vi "test_DELETE.vi"(11 "NXT":T1={"Hardware"="NXT", "Flattened String"=""}) -> (0 "right(T)/left(F)":bool)   [LabVIEW 2012]
uses:
  <vilib>/NXT/Subs/LVHSConnector.ctl
  <vilib>/NXT/Subs/MotorOutput.ctl
  <vilib>/NXT/Block Support/NXT_InputPort.ctl
  <vilib>/NXT/Dual Mode Library/Motors/MotorOn.vi
  <vilib>/NXT/Dual Mode Library/Motors/MotorReverse.vi
  <vilib>/NXT/Dual Mode Library/Motors/MotorBrake.vi
  <vilib>/NXT/Dual Mode Library/Display/clearDisplay.vi
  <vilib>/NXT/Dual Mode Library/Waits/Wait_Num(msec).vi
  <vilib>/NXT/Dual Mode Library/Sound/Tone.vi
  <vilib>/NXT/Dual Mode Library/Display/drawLine.vi
  <vilib>/NXT/Dual Mode Library/prims/addArrayElements_int.vi
  <vilib>/NXT/Dual Mode Library/prims/rotateArray/rotateArray_int.vi
  <vilib>/NXT/Dual Mode Library/Waits/Wait_Num.vi
  <vilib>/NXT/Dual Mode Library/Display/drawText.vi
  <vilib>/NXT/Dual Mode Library/Display/drawNumber.vi
panel:
  in  "degrees to  rotate":dbl
  out "Array 2":i32[](array[numeric])
types:
  T1 = typedef "LVHSConnector.ctl" = cluster{"Hardware":string, "Flattened String":string}
  T2 = typedef "MotorOutput.ctl" = u8
  T3 = typedef "NXT_InputPort.ctl" = u8
  T4 = cluster{"x-y*floor(x/y)":i32, "Start X":i16, "x-y*floor(x/y)":i32, i16}
  T5 = cluster{"x":i32, "Start X":i16, "x":i32, "Start X":i16}
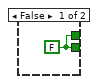
[diagram p2: hidden frame]
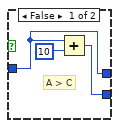
[diagram p3: hidden frame]
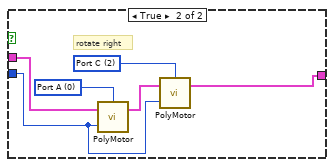
[diagram p5: hidden frame]
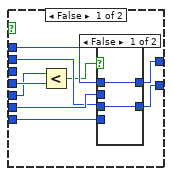
[diagram p16: hidden frame]
diagram:
  w6 = 0
  w9 = T2 5 items=["Port A"=0, "Port B"=1, "Port C"=2, "Ports A & B"=4, "Ports A & C"=5, "Ports B & C"=6, "All Ports"=3] ("Output Port (All Ports)")
  w7 = T2 5 items=["Port A"=0, "Port B"=1, "Port C"=2, "Ports A & B"=4, "Ports A & C"=5, "Ports B & C"=6, "All Ports"=3] ("Output Port (All Ports)")
  w16 = T2 5 items=["Port A"=0, "Port B"=1, "Port C"=2, "Ports A & B"=4, "Ports A & C"=5, "Ports B & C"=6, "All Ports"=3] ("Port (All Ports)")
  w3 = i16 100 ("y")
  (unwired) 2.09 ("Max Value")
  w21 = T2 5 items=["Port A"=0, "Port B"=1, "Port C"=2, "Ports A & B"=4, "Ports A & C"=5, "Ports B & C"=6, "All Ports"=3] ("Port (All Ports)")
  w25 = T2 5 items=["Port A"=0, "Port B"=1, "Port C"=2, "Ports A & B"=4, "Ports A & C"=5, "Ports B & C"=6, "All Ports"=3] ("Port (All Ports)")
  w32 = T2 5 items=["Port A"=0, "Port B"=1, "Port C"=2, "Ports A & B"=4, "Ports A & C"=5, "Ports B & C"=6, "All Ports"=3] ("Port (All Ports)")
  w38 = T2 5 items=["Port A"=0, "Port B"=1, "Port C"=2, "Ports A & B"=4, "Ports A & C"=5, "Ports B & C"=6, "All Ports"=3] ("Port (All Ports)")
  w42 = T2 2 items=["Port A"=0, "Port B"=1, "Port C"=2, "Ports A & B"=4, "Ports A & C"=5, "Ports B & C"=6, "as"=3] ("Output Port (All Ports)")
  w40 = T2 0 items=["Port A"=0, "Port B"=1, "Port C"=2, "Ports A & B"=4, "Ports A & C"=5, "Ports B & C"=6, "as"=3] ("Output Port (All Ports)")
  (unwired) 6.283185307179586 ("Pi Multiplied By 2")
  w60 = i16 -1 ("Start X")
  (unwired) FALSE
  w26 = TRUE
  w37 = 40 ("Power (75)")
  # "Drive forward in a stright line.\nStop if:\n distance to wall is less then X.\n one of the wheels stops rotating"
  # "rotations"
  # "motor C"
  # "motor A"
  # "2.09 for Nicks robot"
  # "ResetMotor.vithe rotate vi also does this,\nbut it does not work unless also done here"
  # "rotate left"
  # "sweep sensor left"
  # "move sensor back"
  # "if sample angle is > 180, rotate right instead of left"
  # "TODO: pass array length to  find paths"
  # "TODO: pass array size to display array vi"
  # "TODO: pass array length to filter & smooth"
  # "number of distance samples"
  # "degrees"
  # "display chosen location"
  # "display list of areas"
  # "if index > 50;\n  test_index  =  100-index\n\nif current_area <  min_area:\n   if  area > current_area:\n     current_area = area\n     current_index = index\nif current_area >=  min_area:\n\n  if test_index < current_index:\n    current_area = area\n    current_index = index"
  # "morgan stanly analysist internship"
  # "minumum candedata size"
  # "find the closest turn candedate to the forward faceing direction with area over a given minimum\nor the largest if non over the minimum are found"
  # "TODO:  min distance considered, min area"
  # "msecs between distance sampling"
  # "motor power level (for scanning)"
  # "TODO: seprate as a vi"
  # "TODO:\n\n combine first and last path condidates (occuring at beginning and end of array-->should be done in the 'find paths' vi\n            \n should have minimum area, take the first one on the left(then right) side that is large enough\n\n     while current_area is less then minimum area:\n            if test_area is greator then current_area:\n                  current_area = test_area\n\ndetermindegress to turn\n\nturn, move forward until some distance is meet (?)"
  # "right max"
  # "left max"
  # "display path candedates"
  # "area"
  # "location"
  # "debug"
  # "screen: 99x63"
  n1 = while {
    stop <- FALSE stop-if-true
    w85 = T2 5 items=["Port A"=0, "Port B"=1, "Port C"=2, "Ports A & B"=4, "Ports A & C"=5, "Ports B & C"=6, "All Ports"=3] ("Port (All Ports)")
    # "ResetMotor.vithe rotate vi also does this,\nbut it does not work unless also done here"
    n2 = call "find_new_direction.vi"() -> ("right(T)/left(F)"=w82:bool, "angle"=w83:dbl, "NXT 2"=w75:T1)  [unwired: 9 in]
    n3 = call <vilib>:"ResetMotor.vi"("NXT"=w75, "Port (All Ports)"=w85) -> ("NXT"=w84:T1)  [unwired: 2 in]
    n4 = call "rotate.vi"("degrees to  rotate"=w83, "right(T)/left(F)"=w82, "power"=u16 75, "NXT 2"=w84) -> ("NXT"=w81:T1)  [unwired: 7 in]
    n5 = call "drive_forward.vi"("min distance"=u16 30 ("power"), "power"=u16 60, "NXT"=w81) -> ("stuck"=w77:bool, "NXT 2"=w76:T1)  [unwired: 7 in]
    n6 = case shown="True" w77 {
      tunnel: w76 -> [w86 w91]
      tunnel: [w86 w88] -> _
      frame False {
      }
      frame True {
        w87 = T2 5 items=["Port A"=0, "Port B"=1, "Port C"=2, "Ports A & B"=4, "Ports A & C"=5, "Ports B & C"=6, "All Ports"=3] ("Output Port (All Ports)")
        # "robot is stuck"
        n7 = call-poly <vilib>:"PolySound.vi"("NXT"=w91) -> ("NXT"=w90:T1)  [unwired: 3 in]
        n8 = call <vilib>:"MotorDistance.vi"("Angle of Rotation (360)"=90, "NXT"=w90, "Output Port (All Ports)"=w87) -> ("NXT"=w88:T1)  [unwired: 1 in]
      }
    }
  }
  n9 = call <vilib>:"ResetMotor.vi"("NXT"="NXT", "Port (All Ports)"=w38) -> ("NXT"=w39:T1)  [unwired: 2 in]
  n10 = call-poly <vilib>:"PolyMotor.vi"("Power (75)"=w37, "NXT"=w39, "Output Port (All Ports)"=w40) -> ("NXT"=w41:T1)  [unwired: 1 in]
  n11 = call-poly <vilib>:"PolyMotor.vi"("Power (75)"=w37, "NXT"=w41, "Output Port (All Ports)"=w42) -> ("NXT"=w36:T1)  [unwired: 1 in]
  n12 = Multiply(x=360.0 ("Max Value"), y=1.45 ("Max Value")) -> (x*y=w33:dbl)
  n13 = while {
    shift-right: [w113] -> w49
    shift-left: i16[] [] -> [w114]
    tunnel: [w110] -> w31
    tunnel: w26 -> [w109]
    tunnel: 5 -> [w106]
    tunnel: w36 -> [w95]
    tunnel: w33 -> [w92]
    i -> [w107]
    stop <- w93 stop-if-true
    w103 = T2 2 items=["Port A"=0, "Port B"=1, "Port C"=2, "Ports A & B"=4, "Ports A & C"=5, "Ports B & C"=6, "as"=3] ("Output Port (All Ports)")
    w104 = T2 0 items=["Port A"=0, "Port B"=1, "Port C"=2, "Ports A & B"=4, "Ports A & C"=5, "Ports B & C"=6, "as"=3] ("Output Port (All Ports)")
    w115 = T3 3 items=["Port 1", "Port 2", "Port 3", "Port 4"] ("Port (Port 4)")
    n14 = call <vilib>:"Rotation.vi"("NXT"=w95, "Port (Port A)"=w104) -> ("Angle of Rotation"=w102:i32, "NXT"=w105:T1)  [unwired: 1 in]
    n15 = call <vilib>:"Rotation.vi"("NXT"=w105, "Port (Port A)"=w103) -> ("Angle of Rotation"=w101:i32, "NXT"=w94:T1)  [unwired: 1 in]
    n16 = Absolute Value(x=w101) -> (abs(x)=w99:i32)
    n17 = Absolute Value(x=w102) -> (abs(x)=w100:i32)
    n18 = Add(x=w99, y=w100) -> (x+y=w98:i32)
    n19 = call <vilib>:"Sonar_cm.vi"("NXT"=w94, "Port (Port 4)"=w115) -> ("Distance (cm)"=w108:i16, "NXT"=w112:T1)  [unwired: 1 in]
    n20 = call-poly <vilib>:"PolyWait.vi"("Time (100 msec)"=w106, "NXT"=w112) -> ("NXT"=w111:T1)  [unwired: 2 in]
    n21 = Divide(x=w98, y=2) -> (x/y=w96:dbl)
    n22 = Greater Or Equal?(x=w96, y=w92) -> (x >= y?=w93:bool)
    n23 = case shown="True" w109 {
      tunnel: w111 -> [w116 w126]
      tunnel: [w116 w127] -> w110
      tunnel: w108 -> [_ w125]
      tunnel: w107 -> [_ w118]
      frame False {
      }
      frame True {
        n24 = call <vilib>:"quot_Remain.vi"("y"=i16 99 ("Start X"), "x"=w118) -> ("x-y*floor(x/y)"=w119:i32)  [unwired: 1 out]
        n25 = Divide(x=i16 60 ("Start X"), y=i16 255 ("Start X")) -> (x/y=w123:dbl)
        n26 = Multiply(x=w125, y=w123) -> (x*y=w128:dbl)
        n27 = To Word Integer(number=w128) -> (16bit integer=w120:i16)
        n28 = Bundle("x-y*floor(x/y)"=w119, "Start X"=i16 0, "x-y*floor(x/y)"=w119, w120) -> (w121:T4)  [unwired: 1 in]
        n29 = call-poly <vilib>:"PolyDisplay.vi"("Line Parameters"=w121, "NXT"=w126) -> ("NXT"=w127:T1)  [unwired: 2 in]
      }
    }
    n30 = Build Array (concatenate)(w114, w108) -> (w113:i16[])
  }
  n31 = Array Size(array=w49) -> (size(s)=w51:i32)
  n32 = call-poly <vilib>:"PolyMotor.vi"("NXT"=w31, "Port (All Ports)"=w32) -> ("NXT"=w28:T1)  [unwired: 2 in]
  n33 = case shown="True" w26 {
    tunnel: w28 -> [w130 w131]
    tunnel: [w130 w131] -> w27
    frame False {
    }
    frame True {
      n34 = Wait (ms)(milliseconds to wait=u32 5000) -> ()  [unwired: 1 out]
    }
  }
  n35 = stacked-sequence {
    tunnel: w49 -> [w137]
    tunnel: [w133] -> w72
    tunnel: w27 -> [w146]
    tunnel: [w146] -> w50
    frame #0 {
      # "array length"
      n36 = Array Subset(array=w137, index=0, length=3 ("index")) -> (w140:i16[])
      n37 = Build Array (concatenate)(w137, w140) -> (w139:i16[])
      n38 = Array Size(array=w139) -> (size(s)=w144:i32)
      n39 = Subtract(x=w144, y=3) -> (x-y=w138:i32)
      n40 = for {
        N: w138 -> [_]
        tunnel: w139 -> [w284]
        shift-right: [w285] -> w134
        shift-left: i32[] [] -> [w286]
        tunnel: w138 -> [w289]
        tunnel: w137 -> [w283]
        i -> [w290]
        w291 = 255
        w298 = 1
        n41 = Add(x=w290, y=w298) -> (x+y=w297:i32)
        n42 = Index Array(array=w284, index=w290) -> (element=w288:i16)
        n43 = Equal?(x=w291, y=w288) -> (x = y?=w295:bool)
        n44 = Add(x=w297, y=w298) -> (x+y=w296:i32)
        n45 = Index Array(array=w284, index=w297) -> (element=w294:i16)
        n46 = Add(x=w296, y=w298) -> (x+y=w299:i32)
        n47 = Index Array(array=w284, index=w296) -> (element=w293:i16)
        n48 = Index Array(array=w284, index=w299) -> (element=w292:i16)
        n49 = case shown="True" w295 {
          tunnel: w294 -> [_ w311]
          tunnel: w293 -> [_ w312]
          tunnel: w292 -> [_ w313]
          tunnel: w291 -> [_ w305]
          tunnel: w290 -> [_ w304]
          tunnel: w289 -> [_ w303]
          tunnel: [w300 w302] -> w287
          tunnel: w288 -> [w300 _]
          tunnel: w283 -> [_ w301]
          frame False {
          }
          frame True {
            n50 = Equal?(x=w305, y=w313) -> (x = y?=w307:bool)
            n51 = Equal?(x=w305, y=w312) -> (x = y?=w309:bool)
            n52 = Equal?(x=w305, y=w311) -> (x = y?=w310:bool)
            n53 = And(x=w310, y=w309) -> (x .and. y?=w308:bool)
            n54 = And(x=w308, y=w307) -> (x .and. y?=w306:bool)
            n55 = case shown="False" w306 {
              tunnel: w305 -> [_ w370]
              tunnel: [w332 w370] -> w302
              tunnel: w304 -> [w315 _]
              tunnel: w303 -> [w316 _]
              tunnel: w301 -> [w317 _]
              frame False {
                w314 = 3 ("length around index")
                # "len around ind."
                # "array"
                # "index"
                # "return a new array of values around an index in an array treated as a ring"
                # "average surounding values != 255"
                n56 = Subtract(x=w316, y=w314) -> (x-y=w328:i32)
                n57 = Less?(x=w315, y=w314) -> (x < y?=w330:bool)
                n58 = Greater Or Equal?(x=w315, y=w328) -> (x >= y?=w327:bool)
                n59 = Or(x=w327, y=w330) -> (x .or. y?=w329:bool)
                n60 = case shown="True" w329 {
                  tunnel: w327 -> [_ w346]
                  tunnel: w316 -> [_ w343]
                  tunnel: w314 -> [w338 w340]
                  tunnel: w317 -> [w339 w345]
                  tunnel: w315 -> [w337 w344]
                  tunnel: [w339 w341] -> w324
                  tunnel: [w338 w340] -> w323
                  tunnel: [w337 w342] -> w322
                  frame False {
                    # "in middle of array"
                  }
                  frame True {
                    n61 = case shown="True" w346 {
                      tunnel: w345 -> [w349 w357]
                      tunnel: w344 -> [w351 w356]
                      tunnel: w343 -> [_ w360]
                      tunnel: [w348 w354] -> w342
                      tunnel: w340 -> [w352 _]
                      tunnel: [w347 w353] -> w341
                      frame False {
                        # "index"
                        # "at beginning of array"
                        n62 = Subtract(x=w352, y=w351) -> (x-y=w350:i32)
                        n63 = Add(x=w351, y=w350) -> (x+y=w348:i32)
                        n64 = call-poly <vilib>:"rotateArray_poly.vi"("Array"=w349, "n"=w350) -> ("rotated array"=w347:i32[])
                      }
                      frame True {
                        # "index"
                        # "at end of array"
                        n65 = Subtract(x=w360, y=w356) -> (x-y=w355:i32)
                        n66 = Subtract(x=w356, y=w355) -> (x-y=w354:i32)
                        n67 = Multiply(x=w355, y=-1.0) -> (x*y=w358:dbl)
                        n68 = call-poly <vilib>:"rotateArray_poly.vi"("Array"=w357, "n"=w358) -> ("rotated array"=w353:i32[])
                      }
                    }
                  }
                }
                n69 = Subtract(x=w322, y=w323) -> (x-y=w325:i32)
                n70 = Add(x=1, y=w322) -> (x+y=w321:i32)
                n71 = Array Subset(array=w324, index=w325, length=w323) -> (w320:i32[])
                n72 = Array Subset(array=w324, index=w321, length=w323) -> (w319:i32[])
                n73 = Build Array (concatenate)(w320, w319) -> (w318:i32[])
                n74 = for {
                  tunnel: w318 -> [w363] mode=indexing
                  shift-right: [w362] -> w334
                  shift-left: i32[] [] -> [w361]
                  n75 = Not Equal?(x=255 ("y"), y=w363) -> (x != y?=w365:bool)
                  n76 = case shown="True" w365 {
                    tunnel: w363 -> [_ w369]
                    tunnel: [w366 w368] -> w362
                    tunnel: w361 -> [w366 w367]
                    frame False {
                    }
                    frame True {
                      n77 = Build Array (concatenate)(w367, w369) -> (w368:i32[])
                    }
                  }
                }
                n78 = call-poly <vilib>:"addArrayElements_poly.vi"("Numeric Array"=w334) -> ("Sum"=w336:i32)
                n79 = Array Size(array=w334) -> (size(s)=w335:i32)
                n80 = Divide(x=w336, y=w335) -> (x/y=w333:dbl)
                n81 = To Word Integer(number=w333) -> (16bit integer=w332:i16)
              }
              frame True {
                # "255"
              }
            }
          }
        }
        n82 = Build Array (concatenate)(w286, w287) -> (w285:i32[])
      }
      n83 = Array Size(array=w134) -> (size(s)=w135:i32)
      n84 = for {
        N: w135 -> [_]
        tunnel: w134 -> [w150]
        shift-right: [w203] -> w133
        shift-left: i8[] [] -> [w202]
        tunnel: w135 -> [_]
        tunnel: w135 -> [w149]
        i -> [w148]
        w147 = 1 ("length around index 2")
        # "len around ind."
        # "array"
        # "index"
        # "return a new array of values around an index in an array treated as a ring"
        # "len around ind."
        # "array"
        # "index"
        # "return a new array of values around an index in an array treated as a ring"
        # "len around ind."
        # "array"
        # "index"
        # "return a new array of values around an index in an array treated as a ring"
        n85 = Subtract(x=w149, y=w147) -> (x-y=w173:i32)
        n86 = Subtract(x=w149, y=w147) -> (x-y=w161:i32)
        n87 = Subtract(x=w149, y=w147) -> (x-y=w186:i32)
        n88 = Less?(x=w148, y=w147) -> (x < y?=w175:bool)
        n89 = Less?(x=w148, y=w147) -> (x < y?=w163:bool)
        n90 = Less?(x=w148, y=w147) -> (x < y?=w188:bool)
        n91 = Greater Or Equal?(x=w148, y=w173) -> (x >= y?=w172:bool)
        n92 = Greater Or Equal?(x=w148, y=w161) -> (x >= y?=w160:bool)
        n93 = Greater Or Equal?(x=w148, y=w186) -> (x >= y?=w185:bool)
        n94 = Or(x=w172, y=w175) -> (x .or. y?=w174:bool)
        n95 = Or(x=w160, y=w163) -> (x .or. y?=w162:bool)
        n96 = Or(x=w185, y=w188) -> (x .or. y?=w187:bool)
        n97 = case shown="True" w174 {
          tunnel: w172 -> [_ w237]
          tunnel: w149 -> [_ w234]
          tunnel: w147 -> [w229 w231]
          tunnel: w150 -> [w230 w236]
          tunnel: w148 -> [w228 w235]
          tunnel: [w230 w232] -> w169
          tunnel: [w229 w231] -> w168
          tunnel: [w228 w233] -> w167
          frame False {
            # "in middle of array"
          }
          frame True {
            n98 = case shown="True" w237 {
              tunnel: w236 -> [w240 w248]
              tunnel: w235 -> [w242 w247]
              tunnel: w234 -> [_ w251]
              tunnel: [w239 w245] -> w233
              tunnel: w231 -> [w243 _]
              tunnel: [w238 w244] -> w232
              frame False {
                # "index"
                # "at beginning of array"
                n99 = Subtract(x=w243, y=w242) -> (x-y=w241:i32)
                n100 = Add(x=w242, y=w241) -> (x+y=w239:i32)
                n101 = call-poly <vilib>:"rotateArray_poly.vi"("Array"=w240, "n"=w241) -> ("rotated array"=w238:i32[])
              }
              frame True {
                # "index"
                # "at end of array"
                n102 = Subtract(x=w251, y=w247) -> (x-y=w246:i32)
                n103 = Subtract(x=w247, y=w246) -> (x-y=w245:i32)
                n104 = Multiply(x=w246, y=-1.0) -> (x*y=w249:dbl)
                n105 = call-poly <vilib>:"rotateArray_poly.vi"("Array"=w248, "n"=w249) -> ("rotated array"=w244:i32[])
              }
            }
          }
        }
        n106 = case shown="True" w162 {
          tunnel: w160 -> [_ w213]
          tunnel: w149 -> [_ w210]
          tunnel: w147 -> [w205 w207]
          tunnel: w150 -> [w206 w212]
          tunnel: w148 -> [w204 w211]
          tunnel: [w206 w208] -> w157
          tunnel: [w205 w207] -> w156
          tunnel: [w204 w209] -> w155
          frame False {
            # "in middle of array"
          }
          frame True {
            n107 = case shown="True" w213 {
              tunnel: w212 -> [w216 w224]
              tunnel: w211 -> [w218 w223]
              tunnel: w210 -> [_ w227]
              tunnel: [w215 w221] -> w209
              tunnel: w207 -> [w219 _]
              tunnel: [w214 w220] -> w208
              frame False {
                # "index"
                # "at beginning of array"
                n108 = Subtract(x=w219, y=w218) -> (x-y=w217:i32)
                n109 = Add(x=w218, y=w217) -> (x+y=w215:i32)
                n110 = call-poly <vilib>:"rotateArray_poly.vi"("Array"=w216, "n"=w217) -> ("rotated array"=w214:i32[])
              }
              frame True {
                # "index"
                # "at end of array"
                n111 = Subtract(x=w227, y=w223) -> (x-y=w222:i32)
                n112 = Subtract(x=w223, y=w222) -> (x-y=w221:i32)
                n113 = Multiply(x=w222, y=-1.0) -> (x*y=w225:dbl)
                n114 = call-poly <vilib>:"rotateArray_poly.vi"("Array"=w224, "n"=w225) -> ("rotated array"=w220:i32[])
              }
            }
          }
        }
        n115 = case shown="True" w187 {
          tunnel: w185 -> [_ w261]
          tunnel: w149 -> [_ w258]
          tunnel: w147 -> [w253 w255]
          tunnel: w150 -> [w254 w260]
          tunnel: w148 -> [w252 w259]
          tunnel: [w254 w256] -> w182
          tunnel: [w253 w255] -> w181
          tunnel: [w252 w257] -> w180
          frame False {
            # "in middle of array"
          }
          frame True {
            n116 = case shown="True" w261 {
              tunnel: w260 -> [w264 w272]
              tunnel: w259 -> [w266 w271]
              tunnel: w258 -> [_ w275]
              tunnel: [w263 w269] -> w257
              tunnel: w255 -> [w267 _]
              tunnel: [w262 w268] -> w256
              frame False {
                # "index"
                # "at beginning of array"
                n117 = Subtract(x=w267, y=w266) -> (x-y=w265:i32)
                n118 = Add(x=w266, y=w265) -> (x+y=w263:i32)
                n119 = call-poly <vilib>:"rotateArray_poly.vi"("Array"=w264, "n"=w265) -> ("rotated array"=w262:i32[])
              }
              frame True {
                # "index"
                # "at end of array"
                n120 = Subtract(x=w275, y=w271) -> (x-y=w270:i32)
                n121 = Subtract(x=w271, y=w270) -> (x-y=w269:i32)
                n122 = Multiply(x=w270, y=-1.0) -> (x*y=w273:dbl)
                n123 = call-poly <vilib>:"rotateArray_poly.vi"("Array"=w272, "n"=w273) -> ("rotated array"=w268:i32[])
              }
            }
          }
        }
        n124 = Subtract(x=w167, y=w168) -> (x-y=w170:i32)
        n125 = Add(x=1, y=w167) -> (x+y=w166:i32)
        n126 = Array Subset(array=w169, index=w170, length=w168) -> (w165:i32[])
        n127 = Array Subset(array=w169, index=w166, length=w168) -> (w164:i32[])
        n128 = Build Array (concatenate)(w165, w164) -> ()  [unwired: 1 out]
        n129 = Subtract(x=w155, y=w156) -> (x-y=w158:i32)
        n130 = Subtract(x=w180, y=w181) -> (x-y=w183:i32)
        n131 = Add(x=1, y=w155) -> (x+y=w154:i32)
        n132 = Add(x=1, y=w180) -> (x+y=w179:i32)
        n133 = Array Subset(array=w157, index=w158, length=w156) -> (w153:i32[])
        n134 = Array Subset(array=w157, index=w154, length=w156) -> (w152:i32[])
        n135 = Array Subset(array=w182, index=w179, length=w181) -> (w177:i32[])
        n136 = Array Subset(array=w182, index=w183, length=w181) -> (w178:i32[])
        n137 = Build Array (concatenate)(w153, w152) -> (→"Array 2":i32[])
        n138 = Build Array (concatenate)(w178, w177) -> (w176:i32[])
        n139 = Index Array(array=w150, index=w148) -> (element=w196:i32)
        n140 = Index Array(array=w176, index=0 ("length around index 2")) -> (element=w194:i32)
        n141 = Index Array(array=w176, index=1 ("length around index 2")) -> (element=w195:i32)
        n142 = Greater?(x=w196, y=w194) -> (0:w199:bool)
        n143 = Greater?(x=w196, y=w195) -> (0:w198:bool)
        n144 = Less?(x=w196, y=w194) -> (x < y?=w193:bool)
        n145 = Less?(x=w196, y=w195) -> (x < y?=w192:bool)
        n146 = And(x=w199, y=w198) -> (x .and. y?=w190:bool)
        n147 = And(x=w193, y=w192) -> (x .and. y?=w189:bool)
        n148 = Or(x=w190, y=w189) -> (x .or. y?=w191:bool)
        n149 = case shown="True" w191 {
          tunnel: w196 -> [w276 _]
          tunnel: w194 -> [_ w281]
          tunnel: w195 -> [_ w280]
          tunnel: [w276 w278] -> w197
          frame False {
          }
          frame True {
            n150 = Add(x=w281, y=w280) -> (x+y=w282:i32)
            n151 = Divide(x=w282, y=2) -> (x/y=w279:dbl)
            n152 = To Word Integer(number=w279) -> (16bit integer=w278:i16)
          }
        }
        n153 = Build Array (concatenate)(w202, w197) -> (w203:i32[])
      }
    }
  }
  n154 = case shown="True" w26 {
    tunnel: w50 -> [w372 w386]
    tunnel: w72 -> [w371 w375]
    tunnel: [w372 w373] -> w69
    tunnel: [w371 w375] -> w71
    frame False {
    }
    frame True {
      # "filter and display array"
      n155 = flat-sequence {
        frame #0 {
          n156 = Wait (ms)(milliseconds to wait=u32 5000) -> ()  [unwired: 1 out]
        }
      }
      n157 = call-poly <vilib>:"PolyDisplay.vi"("NXT"=w386) -> ("NXT"=w385:T1)  [unwired: 3 in]
      n158 = Array Size(array=w375) -> (size(s)=w377:i32)
      n159 = Divide(x=w377, y=98) -> (x/y=w379:dbl)
      n160 = Subtract(x=w377, y=10) -> (x-y=w376:i32)
      n161 = call-poly <vilib>:"PolyWait.vi"("Time (1 sec)"=i16 1 ("Start X"), "NXT"=w385) -> ("NXT"=w374:T1)  [unwired: 2 in]
      n162 = Divide(x=i16 60 ("Start X"), y=i16 255 ("Start X")) -> (x/y=w384:dbl)
      n163 = while {
        tunnel: [w388] -> w373
        tunnel: w384 -> [w407]
        tunnel: w374 -> [w404]
        tunnel: w379 -> [w403]
        shift-right: [w398] -> _
        shift-left: 0 -> [w399]
        tunnel: w377 -> [w389]
        tunnel: w375 -> [w392]
        tunnel: w376 -> [w390]
        i -> [w400]
        stop <- w394 stop-if-true
        n164 = Add(x=w399, y=w403) -> (x+y=w398:dbl)
        n165 = To Word Integer(number=w399) -> (16bit integer=w397:i16)
        n166 = Greater?(x=w397, y=w390) -> (0:w393:bool)
        n167 = Greater?(x=w400, y=w389) -> (0:w401:bool)
        n168 = Index Array(array=w392, index=w397) -> (element=w391:i32)
        n169 = Greater?(x=w400, y=99) -> (0:w396:bool)
        n170 = Multiply(x=w391, y=w407) -> (x*y=w409:dbl)
        n171 = Or(x=w396, y=w401) -> (x .or. y?=w395:bool)
        n172 = Or(x=w393, y=w395) -> (x .or. y?=w394:bool)
        n173 = To Word Integer(number=w409) -> (16bit integer=w406:i16)
        n174 = Bundle(w400, "Start X"=i16 0, w400, w406) -> (w405:cluster{i32, "Start X":i16, i32, i16})  [unwired: 1 in]
        n175 = call-poly <vilib>:"PolyDisplay.vi"("Line Parameters"=w405, "NXT"=w404) -> ("NXT"=w388:T1)  [unwired: 2 in]
      }
    }
  }
  n176 = call-poly <vilib>:"PolyDisplay.vi"("NXT"=w69) -> ("NXT"=w47:T1)  [unwired: 3 in]
  n177 = stacked-sequence {
    tunnel: w71 -> [w413]
    tunnel: [w411] -> w70
    tunnel: [w412] -> w43
    tunnel: w47 -> [w478]
    tunnel: [w478] -> w46
    frame #0 {
      w441 = FALSE
      w440 = -1 ("x")
      w473 = 2 ("x")
      # "?\nkeep track of \nfirst, last, area\nof the first and\nlast groups (with\nindexes starting\nat 0 or ending at\nthe array max"
      # "dont forget about the last one"
      # "30"
      # "TODO: seporate this as a vi"
      # "position--area  arrau"
      # "start--end--area  array"
      # "combine first and last candedates, if any"
      # "construct position--area array"
      # "start"
      # "in block ?"
      # "area"
      # "next index"
      # "index"
      # "min distance"
      # "found blocks"
      n178 = Array Size(array=w413) -> (size(s)=w443:i32)
      n179 = Subtract(x=w443, y=w473) -> (x-y=w474:i32)
      n180 = Subtract(x=w443, y=1) -> (x-y=w424:i32)
      n181 = Subtract(x=w443, y=2 ("x")) -> (x-y=w476:i32)
      n182 = Array Subset(array=w413, index=w474, length=w473) -> (w470:i32[])
      n183 = Array Subset(array=w413, index=0 ("x"), length=2 ("x")) -> (w475:i32[])
      n184 = Build Array (concatenate)(w475, w413, w470) -> (w463:i32[])
      n185 = Index Array(array=w463, index=2 ("x")) -> (element=w465:i32)
      n186 = Index Array(array=w463, index=3 ("x")) -> (element=w464:i32)
      n187 = Index Array(array=w463, index=1 ("x")) -> (element=w466:i32)
      n188 = for {
        N: w476 -> [_]
        shift-right: [w640] -> _
        shift-left: w466 -> [w663]
        shift-right: [w639] -> _
        shift-left: w465 -> [w640]
        shift-right: [w659] -> _
        shift-left: w464 -> [w639]
        tunnel: w463 -> [w660]
        shift-right: [w658] -> _
        shift-left: 4 ("x") -> [w657]
        tunnel: 65 ("x") -> [w653]
        shift-right: [w649] -> w456
        shift-left: FALSE -> [w652]
        shift-right: [w650] -> w453
        shift-left: 0 ("x") -> [w651]
        shift-right: [w646] -> w455
        shift-left: 0 ("x") -> [w648]
        shift-right: [w643] -> w454
        shift-left: 0 ("x") -> [w647]
        shift-right: [w641] -> w452
        shift-left: i16[] [] -> [w645]
        # "seporate array of distance values into blocks of continuous distances"
        # "average"
        # "c"
        # "b"
        # "a"
        n189 = Add(x=w663, y=w640) -> (x+y=w664:i32)
        n190 = Index Array(array=w660, index=w657) -> (element=w659:i32)
        n191 = Add(x=w657, y=1 ("x")) -> (x+y=w658:i32)
        n192 = Add(x=w664, y=w639) -> (x+y=w662:i32)
        n193 = Divide(x=w662, y=3 ("x")) -> (x/y=w654:dbl)
        n194 = Greater?(x=w654, y=w653) -> (0:w655:bool)
        n195 = case shown="False" w655 {
          tunnel: w652 -> [w674 w695]
          tunnel: w651 -> [w669 w698]
          tunnel: w639 -> [_ w697]
          tunnel: [w668 w696] -> w650
          tunnel: [w673 w694] -> w649
          tunnel: w648 -> [w671 w693]
          tunnel: w647 -> [w670 w692]
          tunnel: [w666 w691] -> w646
          tunnel: w645 -> [w672 w689]
          tunnel: [w667 w690] -> w644
          tunnel: [w665 w688] -> w641
          frame False {
            n196 = case shown="True" w674 {
              selector: w674 -> [w677 _]
              tunnel: [w677 FALSE] -> w673
              tunnel: w672 -> [w679 w686]
              tunnel: w671 -> [w675 w681]
              tunnel: w670 -> [w676 w682]
              tunnel: w669 -> [w678 w683]
              tunnel: [w678 w683] -> w668
              tunnel: [w676 w682] -> w667
              tunnel: [w675 w681] -> w666
              tunnel: [w679 w680] -> w665
              frame False {
              }
              frame True {
                # "area"
                # "end"
                # "start"
                # "end of block"
                n197 = Build Array (concatenate)(w686, w681) -> (w685:i32[])
                n198 = Build Array (concatenate)(w685, w682) -> (w684:i32[])
                n199 = Build Array (concatenate)(w684, w683) -> (w680:i32[])
              }
            }
          }
          frame True {
            n200 = case shown="False" w695 {
              tunnel: w698 -> [_ w709]
              tunnel: w697 -> [w699 w708]
              tunnel: [w699 w707] -> w696
              tunnel: w695 -> [_ w706]
              tunnel: [TRUE w706] -> w694
              tunnel: w693 -> [_ w705]
              tunnel: w692 -> [w701 w704]
              tunnel: [w701 w705] -> w691
              tunnel: [w701 w704] -> w690
              tunnel: w689 -> [w700 w703]
              tunnel: [w700 w703] -> w688
              frame False {
                # "block start"
              }
              frame True {
                # "in block"
                n201 = Add(x=w708, y=w709) -> (x+y=w707:i32)
              }
            }
          }
        }
        n202 = Add(x=w644, y=1 ("x")) -> (x+y=w643:i32)
      }
      n203 = case shown="True" w456 {
        tunnel: w455 -> [_ w636]
        tunnel: w454 -> [_ w633]
        tunnel: w453 -> [_ w632]
        tunnel: [w629 w631] -> w411
        tunnel: w452 -> [w629 w630]
        frame False {
        }
        frame True {
          # "area"
          # "end"
          # "start"
          n204 = Build Array (concatenate)(w630, w636) -> (w637:i32[])
          n205 = Add(x=w633, y=1 ("x")) -> (x+y=w634:i32)
          n206 = Build Array (concatenate)(w637, w634) -> (w638:i32[])
          n207 = Build Array (concatenate)(w638, w632) -> (w631:i32[])
        }
      }
      n208 = Array Size(array=w411) -> (size(s)=w450:i32)
      n209 = Divide(x=w450, y=3) -> (x/y=w448:dbl)
      n210 = To Word Integer(number=w448) -> (16bit integer=w447:i16)
      n211 = for {
        N: w447 -> [_]
        tunnel: w411 -> [w567]
        shift-right: [w548] -> w427
        shift-left: w440 -> [w560]
        shift-right: [w547] -> w428
        shift-left: w440 -> [w559]
        shift-right: [w546] -> w429
        shift-left: w440 -> [w558]
        shift-right: [w553] -> w430
        shift-left: w440 -> [w557]
        shift-right: [w551] -> w431
        shift-left: w440 -> [w556]
        shift-right: [w549] -> w432
        shift-left: w440 -> [w555]
        shift-right: [w568] -> _
        shift-left: 0 ("x") -> [w554]
        shift-right: [w569] -> _
        shift-left: 1 ("x") -> [w552]
        shift-right: [w570] -> _
        shift-left: 2 ("x") -> [w550]
        tunnel: w424 -> [w561]
        shift-right: [w542] -> w436
        shift-left: w441 -> [w544]
        shift-right: [w543] -> w437
        shift-left: w441 -> [w545]
        shift-right: [w540] -> w426
        shift-left: i16[] [] -> [w541]
        w566 = 3 ("x")
        n212 = Index Array(array=w567, index=w552) -> (element=w538:i32)
        n213 = Index Array(array=w567, index=w554) -> (element=w537:i32)
        n214 = Index Array(array=w567, index=w550) -> (element=w539:i32)
        n215 = Equal?(x=w538, y=w561) -> (x = y?=w565:bool)
        n216 = Add(x=w550, y=w566) -> (x+y=w570:i32)
        n217 = Add(x=w566, y=w552) -> (x+y=w569:i32)
        n218 = Add(x=w566, y=w554) -> (x+y=w568:i32)
        n219 = Equal?(x=w537, y=0 ("x")) -> (x = y?=w562:bool)
        n220 = Or(x=w562, y=w565) -> (x .or. y?=w564:bool)
        n221 = case shown="False" w564 {
          tunnel: w562 -> [_ w610]
          tunnel: w560 -> [w588 w609]
          tunnel: w559 -> [w587 w608]
          tunnel: w558 -> [w586 w607]
          tunnel: w557 -> [w585 w606]
          tunnel: w556 -> [w584 w605]
          tunnel: w555 -> [w583 w604]
          tunnel: w537 -> [w575 w603]
          tunnel: [w585 w602] -> w553
          tunnel: w538 -> [w576 w601]
          tunnel: [w584 w600] -> w551
          tunnel: w539 -> [w580 w599]
          tunnel: [w583 w598] -> w549
          tunnel: [w588 w597] -> w548
          tunnel: [w587 w596] -> w547
          tunnel: [w586 w595] -> w546
          tunnel: w545 -> [w582 w594]
          tunnel: w544 -> [w581 w593]
          tunnel: [w581 w592] -> w542
          tunnel: [w582 w591] -> w543
          tunnel: w541 -> [w571 w590]
          tunnel: [w579 w589] -> w540
          frame False {
            # "position"
            # "area"
            n222 = Add(x=w575, y=w576) -> (x+y=w578:i32)
            n223 = Divide(x=w578, y=2 ("x")) -> (x/y=w574:dbl)
            n224 = To Word Integer(number=w574) -> (16bit integer=w573:i16)
            n225 = Build Array (concatenate)(w571, w573) -> (w572:i32[])
            n226 = Build Array (concatenate)(w572, w580) -> (w579:i32[])
          }
          frame True {
            n227 = case shown="True" w610 {
              tunnel: w609 -> [w613 _]
              tunnel: w608 -> [w612 _]
              tunnel: w607 -> [w611 _]
              tunnel: w606 -> [_ w625]
              tunnel: w605 -> [_ w624]
              tunnel: w604 -> [_ w623]
              tunnel: w603 -> [w619 w628]
              tunnel: [w619 w625] -> w602
              tunnel: w601 -> [w618 w627]
              tunnel: [w618 w624] -> w600
              tunnel: w599 -> [w617 w626]
              tunnel: [w617 w623] -> w598
              tunnel: [w613 w628] -> w597
              tunnel: [w612 w627] -> w596
              tunnel: [w611 w626] -> w595
              tunnel: w594 -> [w615 _]
              tunnel: w593 -> [_ w622]
              tunnel: [TRUE w622] -> w592
              tunnel: [w615 TRUE] -> w591
              tunnel: w590 -> [w614 w620]
              tunnel: [w614 w620] -> w589
              frame False {
                # "found last"
              }
              frame True {
                # "found first"
              }
            }
          }
        }
      }
      n228 = And(x=w437, y=w436) -> (x .and. y?=w438:bool)
      n229 = case shown="True" w438 {
        tunnel: [w517 w536] -> w435
        tunnel: [w516 w536] -> w434
        tunnel: w437 -> [w517 _]
        tunnel: w436 -> [w516 _]
        tunnel: w432 -> [w514 w531]
        tunnel: w431 -> [w513 w527]
        tunnel: w430 -> [w512 w526]
        tunnel: w429 -> [w511 w532]
        tunnel: w428 -> [w510 w528]
        tunnel: w427 -> [w509 _]
        tunnel: w426 -> [w515 w530]
        tunnel: [w515 w534] -> w425
        tunnel: w424 -> [_ w524]
        tunnel: [w514 w522] -> w418
        tunnel: [w513 w522] -> w419
        tunnel: [w512 w522] -> w420
        tunnel: [w511 w522] -> w421
        tunnel: [w510 w522] -> w422
        tunnel: [w509 w522] -> w423
        frame False {
        }
        frame True {
          w522 = -1 ("x")
          w536 = FALSE
          # "area"
          # "pos"
          # "append first and last arrays"
          n230 = Subtract(x=w527, y=w526) -> (x-y=w529:i32)
          n231 = Add(x=w532, y=w531) -> (x+y=w533:i32)
          n232 = Add(x=w528, y=w529) -> (x+y=w520:i32)
          n233 = Divide(x=w520, y=2 ("x")) -> (x/y=w519:dbl)
          n234 = To Word Integer(number=w519) -> (16bit integer=w518:i16)
          n235 = Add(x=w518, y=w526) -> (x+y=w525:i32)
          n236 = call <vilib>:"quot_Remain.vi"("y"=w524, "x"=w525) -> ("x-y*floor(x/y)"=w523:i32)  [unwired: 1 out]
          n237 = Build Array (concatenate)(w530, w523) -> (w535:i32[])
          n238 = Build Array (concatenate)(w535, w533) -> (w534:i32[])
        }
      }
      n239 = case shown="True" w435 {
        tunnel: w434 -> [w494 w508]
        tunnel: [w494 w508] -> w433
        tunnel: w425 -> [w493 w499]
        tunnel: w423 -> [_ w502]
        tunnel: w422 -> [_ w503]
        tunnel: w421 -> [_ w500]
        tunnel: w420 -> [w490 w495]
        tunnel: w419 -> [w491 w496]
        tunnel: w418 -> [w492 w497]
        tunnel: [w493 w498] -> w417
        tunnel: [w492 w497] -> w414
        tunnel: [w491 w496] -> w415
        tunnel: [w490 w495] -> w416
        frame False {
        }
        frame True {
          # "area"
          # "pos"
          # "add first"
          n240 = Add(x=w502, y=w503) -> (x+y=w505:i32)
          n241 = Divide(x=w505, y=2 ("x")) -> (x/y=w507:dbl)
          n242 = To Word Integer(number=w507) -> (16bit integer=w501:i16)
          n243 = Build Array (concatenate)(w499, w501) -> (w504:i32[])
          n244 = Build Array (concatenate)(w504, w500) -> (w498:i32[])
        }
      }
      n245 = case shown="True" w433 {
        tunnel: w417 -> [w479 w485]
        tunnel: w416 -> [_ w484]
        tunnel: w415 -> [_ w483]
        tunnel: w414 -> [_ w482]
        tunnel: [w479 w480] -> w412
        frame False {
        }
        frame True {
          # "area"
          # "pos"
          # "add last"
          n246 = Add(x=w484, y=w483) -> (x+y=w489:i32)
          n247 = Divide(x=w489, y=2 ("x")) -> (x/y=w487:dbl)
          n248 = To Word Integer(number=w487) -> (16bit integer=w481:i16)
          n249 = Build Array (concatenate)(w485, w481) -> (w486:i32[])
          n250 = Build Array (concatenate)(w486, w482) -> (w480:i32[])
        }
      }
    }
  }
  n251 = Array Size(array=w43) -> (size(s)=w44:i32)
  n252 = case shown="True" w26 {
    tunnel: w70 -> [w710 w727]
    tunnel: w46 -> [w711 w725]
    tunnel: [w711 w726] -> w65
    tunnel: w71 -> [_ w728]
    tunnel: [w710 w724] -> _
    frame False {
    }
    frame True {
      n253 = stacked-sequence {
        tunnel: w728 -> [w764]
        tunnel: [w763] -> w714
        tunnel: w727 -> [w753]
        tunnel: w725 -> [w754]
        tunnel: [w754] -> w713
        tunnel: [w753] -> w724
        frame #0 {
          # "end"
          n254 = Array Size(array=w753) -> (size(s)=w757:i32)
          n255 = Divide(x=w757, y=3) -> (x/y=w755:dbl)
          n256 = for {
            N: w755 -> [_]
            shift-right: [w784] -> _
            shift-left: i16 0 ("Start X") -> [w781]
            shift-right: [w783] -> _
            shift-left: i16 1 ("Start X") -> [w780]
            shift-right: [w772] -> w762
            shift-left: i16[] [] -> [w774]
            tunnel: w753 -> [w779]
            shift-right: [w777] -> w759
            shift-left: i16 0 ("Start X") -> [w778]
            w785 = 3 ("y")
            # "end"
            # "start"
            n257 = Index Array(array=w779, index=w780) -> (element=w777:i32)
            n258 = Index Array(array=w779, index=w781) -> (element=w776:i32)
            n259 = Add(x=w781, y=w785) -> (x+y=w784:i32)
            n260 = Subtract(x=w777, y=w776) -> (x-y=w775:i32)
            n261 = Subtract(x=w776, y=w778) -> (x-y=w782:i32)
            n262 = Add(x=w780, y=w785) -> (x+y=w783:i32)
            n263 = for {
              N: w782 -> [_]
              shift-right: [w790] -> w773
              shift-left: w774 -> [w791]
              n264 = Build Array (concatenate)(w791, i16 0 ("Start X")) -> (w790:i16[])
            }
            n265 = for {
              N: w775 -> [_]
              shift-right: [w786] -> w772
              shift-left: w773 -> [w787]
              n266 = Build Array (concatenate)(w787, i16 1 ("Start X")) -> (w786:i16[])
            }
          }
          n267 = Subtract(x=i16 99 ("Start X"), y=w759) -> (x-y=w758:i32)
          n268 = for {
            N: w758 -> [_]
            shift-right: [w770] -> w761
            shift-left: w762 -> [w771]
            n269 = Build Array (concatenate)(w771, i16 0 ("Start X")) -> (w770:i16[])
          }
          n270 = Multiply(x=w761, y=w764) -> (x*y=w763:i32[])
        }
      }
      n271 = Array Size(array=w714) -> (size(s)=w716:i32)
      n272 = Divide(x=w716, y=98) -> (x/y=w718:dbl)
      n273 = Subtract(x=w716, y=10) -> (x-y=w715:i32)
      n274 = Divide(x=i16 60 ("Start X"), y=i16 255 ("Start X")) -> (x/y=w723:dbl)
      n275 = while {
        tunnel: [w729] -> w712
        tunnel: w723 -> [w748]
        tunnel: w713 -> [w745]
        tunnel: w718 -> [w744]
        shift-right: [w739] -> _
        shift-left: 0 -> [w740]
        tunnel: w716 -> [w730]
        tunnel: w714 -> [w733]
        tunnel: w715 -> [w731]
        i -> [w741]
        stop <- w735 stop-if-true
        n276 = Add(x=w740, y=w744) -> (x+y=w739:dbl)
        n277 = To Word Integer(number=w740) -> (16bit integer=w738:i16)
        n278 = Greater?(x=w738, y=w731) -> (0:w734:bool)
        n279 = Greater?(x=w741, y=w730) -> (0:w742:bool)
        n280 = Index Array(array=w733, index=w738) -> (element=w732:i32)
        n281 = Greater?(x=w741, y=99) -> (0:w737:bool)
        n282 = Or(x=w737, y=w742) -> (x .or. y?=w736:bool)
        n283 = Multiply(x=w732, y=w748) -> (x*y=w750:dbl)
        n284 = Or(x=w734, y=w736) -> (x .or. y?=w735:bool)
        n285 = To Word Integer(number=w750) -> (16bit integer=w747:i16)
        n286 = Bundle(w741, "Start X"=i16 0, w741, w747) -> (w746:cluster{i32, "Start X":i16, i32, i16})  [unwired: 1 in]
        n287 = call-poly <vilib>:"PolyDisplay.vi"("Line Parameters"=w746, "NXT"=w745) -> ("NXT"=w729:T1)  [unwired: 2 in]
      }
      n288 = stacked-sequence {
        tunnel: [_ w751] -> w726
        tunnel: w712 -> [_ w751]
        frame #0 {
        }
        frame #1 {
          n289 = Wait (ms)(milliseconds to wait=u32 5000) -> ()  [unwired: 1 out]
        }
      }
    }
  }
  n290 = Divide(x=w44, y=i16 2 ("Start X")) -> (x/y=w66:dbl)
  n291 = To Byte Integer(number=w66) -> (8bit integer=w64:i8)
  n292 = case shown="True" w26 {
    tunnel: w65 -> [w792 w801]
    tunnel: w43 -> [_ w795]
    tunnel: [w792 w794] -> w63
    frame False {
    }
    frame True {
      # "0 for list of positions"
      n293 = Array Size(array=w795) -> (size(s)=w799:i32)
      n294 = Divide(x=w799, y=2) -> (x/y=w797:dbl)
      n295 = To Word Integer(number=w797) -> (16bit integer=w796:i16)
      n296 = for {
        N: w796 -> [_]
        tunnel: w801 -> [w813]
        tunnel: [w813] -> w803
        shift-right: [w814] -> w802
        shift-left: "" ("Text") -> [w816]
        shift-right: [w811] -> _
        shift-left: i16 1 ("Start X") -> [w809]
        tunnel: w795 -> [w808]
        n297 = Index Array(array=w808, index=w809) -> (element=w807:i32)
        n298 = Add(x=w809, y=i16 2 ("Start X")) -> (x+y=w811:i16)
        n299 = call <vilib>:"NXT_floatToString.vi"("number"=w807) -> ("string"=w815:string)
        n300 = Concatenate Strings(w816, " " ("Text"), w815) -> (w814:string)
      }
      n301 = call-poly <vilib>:"PolyDisplay.vi"("Text"=w802, "NXT"=w803) -> ("NXT"=w793:T1)  [unwired: 2 in]
      n302 = stacked-sequence {
        tunnel: w793 -> [_ w805]
        tunnel: [_ w805] -> w794
        frame #0 {
        }
        frame #1 {
          n303 = Wait (ms)(milliseconds to wait=u32 5000) -> ()  [unwired: 1 out]
        }
      }
    }
  }
  n304 = for {
    N: w64 -> [_]
    tunnel: w43 -> [w838]
    shift-right: [w837] -> _
    shift-left: i16 0 ("Start X") -> [w820]
    shift-right: [w836] -> _
    shift-left: i16 1 ("Start X") -> [w834]
    shift-right: [w829] -> w48
    shift-left: w60 -> [w824]
    shift-right: [w828] -> w59
    shift-left: w60 -> [w821]
    tunnel: w63 -> [w833]
    tunnel: i16 700 ("Start X") -> [w822]
    tunnel: [w833] -> w56
    tunnel: w51 -> [w818]
    w835 = i16 2 ("Start X")
    # "area"
    # "position"
    n305 = Less?(x=w821, y=w822) -> (x < y?=w831:bool)
    n306 = Index Array(array=w838, index=w834) -> (element=w830:i32)
    n307 = Index Array(array=w838, index=w820) -> (element=w823:i32)
    n308 = Divide(x=w818, y=i16 2 ("Start X")) -> (x/y=w817:dbl)
    n309 = Add(x=w820, y=w835) -> (x+y=w837:i16)
    n310 = Add(x=w834, y=w835) -> (x+y=w836:i16)
    n311 = Greater Or Equal?(x=w824, y=w817) -> (x >= y?=w832:bool)
    n312 = Greater Or Equal?(x=w823, y=w817) -> (x >= y?=w826:bool)
    n313 = case shown="True" w832 {
      tunnel: w824 -> [w868 w870]
      tunnel: [w868 w871] -> w827
      tunnel: w818 -> [_ w869]
      frame False {
      }
      frame True {
        n314 = Subtract(x=w869, y=w870) -> (x-y=w871:i32)
      }
    }
    n315 = case shown="True" w826 {
      tunnel: w823 -> [w839 w842]
      tunnel: [w839 w841] -> w825
      tunnel: w818 -> [_ w840]
      frame False {
      }
      frame True {
        n316 = Subtract(x=w840, y=w842) -> (x-y=w841:i32)
      }
    }
    n317 = case shown="True" w831 {
      tunnel: w823 -> [w851 w861]
      tunnel: w830 -> [w850 w859]
      tunnel: [w849 w860] -> w829
      tunnel: [w848 w858] -> w828
      tunnel: w827 -> [w845 _]
      tunnel: w825 -> [w844 _]
      tunnel: w824 -> [w847 w857]
      tunnel: w821 -> [w846 w856]
      tunnel: w821 -> [_ w863]
      frame False {
        n318 = Less?(x=w844, y=w845) -> (x < y?=w843:bool)
        n319 = case shown="False" w843 {
          tunnel: w851 -> [_ w855]
          tunnel: w850 -> [_ w854]
          tunnel: [w853 w855] -> w849
          tunnel: [w852 w854] -> w848
          tunnel: w847 -> [w853 _]
          tunnel: w846 -> [w852 _]
          frame False {
          }
          frame True {
          }
        }
      }
      frame True {
        n320 = Greater?(x=w859, y=w863) -> (0:w862:bool)
        n321 = case shown="True" w862 {
          tunnel: w861 -> [_ w867]
          tunnel: [w864 w867] -> w860
          tunnel: w859 -> [_ w866]
          tunnel: [w865 w866] -> w858
          tunnel: w857 -> [w864 _]
          tunnel: w856 -> [w865 _]
          frame False {
          }
          frame True {
          }
        }
      }
    }
  }
  n322 = Divide(x=w51, y=i16 2 ("Start X")) -> (x/y=w52:dbl)
  n323 = Greater Or Equal?(x=w48, y=w52) -> (x >= y?=w55:bool)
  n324 = Greater Or Equal?(x=w48, y=w52) -> ()  [unwired: 1 out]
  n325 = case shown="True" w26 {
    tunnel: w48 -> [_ w875]
    tunnel: w56 -> [w872 w877]
    tunnel: [w872 w873] -> w24
    tunnel: w59 -> [_ _]
    frame False {
      # "turn right"
    }
    frame True {
      # "turn left"
      n326 = call-poly <vilib>:"PolyDisplay.vi"("number"=w875, "NXT"=w877) -> ("NXT"=w880:T1)  [unwired: 2 in]
      n327 = Bundle("x"=w875, "Start X"=i16 0, "x"=w875, "Start X"=i16 63) -> (w876:T5)  [unwired: 1 in]
      n328 = call-poly <vilib>:"PolyDisplay.vi"("Line Parameters"=w876, "NXT"=w880) -> ("NXT"=w874:T1)  [unwired: 2 in]
      n329 = stacked-sequence {
        tunnel: w874 -> [_ w881]
        tunnel: [_ w881] -> w873
        frame #0 {
        }
        frame #1 {
          n330 = Wait (ms)(milliseconds to wait=u32 5000) -> ()  [unwired: 1 out]
        }
      }
    }
  }
  n331 = case shown="True" w55 {
    tunnel: w48 -> [w883 w884]
    tunnel: [w883 w884] -> w54
    tunnel: w51 -> [_ w885]
    frame False {
    }
    frame True {
      # "test"
      n332 = Subtract(x=w885, y=w884) -> ()  [unwired: 1 out]
    }
  }
  n333 = Divide(x=w54, y=w51) -> (x/y=w57:dbl)
  n334 = Multiply(x=i16 360 ("Start X"), y=w57) -> ()  [unwired: 1 out]
  n335 = call <vilib>:"ResetMotor.vi"("NXT"=w24, "Port (All Ports)"=w25) -> ("NXT"=w12:T1)  [unwired: 2 in]
  n336 = call <vilib>:"ResetMotor.vi"("NXT"=w12, "Port (All Ports)"=w16) -> ("NXT"=w14:T1)  [unwired: 2 in]
  n337 = call-poly <vilib>:"PolyWait.vi"("Time (100 msec)"=i16 100 ("y"), "NXT"=w14) -> ("NXT"=w13:T1)  [unwired: 2 in]
  n338 = case shown="False" FALSE {
    tunnel: u16 75 ("power") -> [w887 w893]
    tunnel: w13 -> [w886 w892]
    tunnel: [w888 w894] -> w23
    frame False {
      w891 = T2 2 items=["Port A"=0, "Port B"=1, "Port C"=2, "Ports A & B"=4, "Ports A & C"=5, "Ports B & C"=6, "as"=3] ("Output Port (All Ports)")
      w889 = T2 0 items=["Port A"=0, "Port B"=1, "Port C"=2, "Ports A & B"=4, "Ports A & C"=5, "Ports B & C"=6, "as"=3] ("Output Port (All Ports)")
      # "rotate left"
      n339 = call-poly <vilib>:"PolyMotor.vi"("Power (75)"=w887, "NXT"=w886, "Output Port (All Ports)"=w889) -> ("NXT"=w890:T1)  [unwired: 1 in]
      n340 = call-poly <vilib>:"PolyMotor.vi"("Power (75)"=w887, "NXT"=w890, "Output Port (All Ports)"=w891) -> ("NXT"=w888:T1)  [unwired: 1 in]
    }
    frame True {
      w897 = T2 2 items=["Port A"=0, "Port B"=1, "Port C"=2, "Ports A & B"=4, "Ports A & C"=5, "Ports B & C"=6, "as"=3] ("Output Port (All Ports)")
      w895 = T2 0 items=["Port A"=0, "Port B"=1, "Port C"=2, "Ports A & B"=4, "Ports A & C"=5, "Ports B & C"=6, "as"=3] ("Output Port (All Ports)")
      # "rotate right"
      n341 = call-poly <vilib>:"PolyMotor.vi"("Power (75)"=w893, "NXT"=w892, "Output Port (All Ports)"=w895) -> ("NXT"=w896:T1)  [unwired: 1 in]
      n342 = call-poly <vilib>:"PolyMotor.vi"("Power (75)"=w893, "NXT"=w896, "Output Port (All Ports)"=w897) -> ("NXT"=w894:T1)  [unwired: 1 in]
    }
  }
  n343 = Multiply(x="degrees to  rotate", y=1.475 ("Max Value")) -> (x*y=w20:dbl)
  n344 = while {
    tunnel: w23 -> [w911]
    tunnel: w20 -> [w901]
    tunnel: [w898] -> w22
    stop <- w899 stop-if-true
    w908 = T2 2 items=["Port A"=0, "Port B"=1, "Port C"=2, "Ports A & B"=4, "Ports A & C"=5, "Ports B & C"=6, "as"=3] ("Output Port (All Ports)")
    w909 = T2 0 items=["Port A"=0, "Port B"=1, "Port C"=2, "Ports A & B"=4, "Ports A & C"=5, "Ports B & C"=6, "as"=3] ("Output Port (All Ports)")
    n345 = call <vilib>:"Rotation.vi"("NXT"=w911, "Port (Port A)"=w909) -> ("Angle of Rotation"=w907:i32, "NXT"=w910:T1)  [unwired: 1 in]
    n346 = Absolute Value(x=w907) -> (abs(x)=w905:i32)
    n347 = call <vilib>:"Rotation.vi"("NXT"=w910, "Port (Port A)"=w908) -> ("Angle of Rotation"=w906:i32, "NXT"=w898:T1)  [unwired: 1 in]
    n348 = Absolute Value(x=w906) -> (abs(x)=w904:i32)
    n349 = Add(x=w904, y=w905) -> (x+y=w903:i32)
    n350 = Divide(x=w903, y=2) -> (x/y=w900:dbl)
    n351 = Greater Or Equal?(x=w900, y=w901) -> (x >= y?=w899:bool)
  }
  n352 = call-poly <vilib>:"PolyMotor.vi"("NXT"=w22, "Port (All Ports)"=w21) -> ("NXT"=w18:T1)  [unwired: 2 in]
  n353 = call-poly <vilib>:"PolyWait.vi"("Time (100 msec)"=w3, "NXT"=w18) -> ("NXT"=w4:T1)  [unwired: 2 in]
  n354 = call <vilib>:"ResetMotor.vi"("NXT"=w4, "Port (All Ports)"=w7) -> ("NXT"=w8:T1)  [unwired: 2 in]
  n355 = while {
    tunnel: w8 -> [w940]
    tunnel: [w927] -> w5
    shift-right: [w921] -> _
    shift-left: w6 -> [w922]
    shift-right: [w917] -> _
    shift-left: w6 -> [w918]
    tunnel: w3 -> [w929]
    tunnel: w3 -> [w925]
    tunnel: [w912] -> w1
    stop <- w915 stop-if-true
    w933 = T2 2 items=["Port A"=0, "Port B"=1, "Port C"=2, "Ports A & B"=4, "Ports A & C"=5, "Ports B & C"=6, "All Ports"=3] ("Output Port (All Ports)")
    w934 = T2 0 items=["Port A"=0, "Port B"=1, "Port C"=2, "Ports A & B"=4, "Ports A & C"=5, "Ports B & C"=6, "All Ports"=3] ("Output Port (All Ports)")
    w935 = T2 2 items=["Port A"=0, "Port B"=1, "Port C"=2, "Ports A & B"=4, "Ports A & C"=5, "Ports B & C"=6, "All Ports"=3] ("Output Port (All Ports)")
    w936 = T2 0 items=["Port A"=0, "Port B"=1, "Port C"=2, "Ports A & B"=4, "Ports A & C"=5, "Ports B & C"=6, "All Ports"=3] ("Output Port (All Ports)")
    w941 = T3 3 items=["Port 1", "Port 2", "Port 3", "Port 4"] ("Port (Port 4)")
    n356 = call <vilib>:"Rotation.vi"("NXT"=w940, "Port (Port A)"=w934) -> ("Angle of Rotation"=w921:i32, "NXT"=w939:T1)  [unwired: 1 in]
    n357 = Equal?(x=w922, y=w921) -> (x = y?=w920:bool)
    n358 = call <vilib>:"Rotation.vi"("NXT"=w939, "Port (Port A)"=w933) -> ("Angle of Rotation"=w917:i32, "NXT"=w938:T1)  [unwired: 1 in]
    n359 = Greater?(x=w917, y=w921) -> ()  [unwired: 1 out]
    n360 = Equal?(x=w918, y=w917) -> (x = y?=w919:bool)
    n361 = Equal?(x=w921, y=w917) -> (x = y?=w932:bool)
    n362 = Or(x=w920, y=w919) -> (x .or. y?=w914:bool)
    n363 = call <vilib>:"Sonar_cm.vi"("NXT"=w938, "Port (Port 4)"=w941) -> ("Distance (cm)"=w930:i16, "NXT"=w931:T1)  [unwired: 1 in]
    n364 = case shown="False" w932 {
      tunnel: [w947 w956] -> w928
      tunnel: w925 -> [w948 w956]
      tunnel: [w946 w956] -> w924
      tunnel: w917 -> [w945 _]
      tunnel: w921 -> [w944 _]
      frame False {
        n365 = Greater?(x=w944, y=w945) -> (0:w949:bool)
        n366 = case shown="True" w949 {
          tunnel: w948 -> [w950 w953]
          tunnel: [w950 w954] -> w947
          tunnel: [w951 w953] -> w946
          frame False {
            # "A > C"
            n367 = Add(x=w950, y=10) -> (x+y=w951:i32)
          }
          frame True {
            # "C > A"
            n368 = Add(x=w953, y=10) -> (x+y=w954:i32)
          }
        }
      }
      frame True {
      }
    }
    n369 = Less Or Equal?(x=w930, y=w929) -> (x <= y?=w916:bool)
    n370 = case shown="True" w914 {
      tunnel: [w942 w943] -> w913
      tunnel: [w942 w943] -> w912
      frame False {
        w942 = FALSE
      }
      frame True {
        w943 = FALSE
      }
    }
    n371 = Or(x=w913, y=w916) -> (x .or. y?=w915:bool)
    n372 = call-poly <vilib>:"PolyMotor.vi"("Power (75)"=w928, "NXT"=w931, "Output Port (All Ports)"=w936) -> ("NXT"=w937:T1)  [unwired: 1 in]
    n373 = call-poly <vilib>:"PolyMotor.vi"("Power (75)"=w924, "NXT"=w937, "Output Port (All Ports)"=w935) -> ("NXT"=w923:T1)  [unwired: 1 in]
    n374 = call-poly <vilib>:"PolyWait.vi"("Time (100 msec)"=100, "NXT"=w923) -> ("NXT"=w927:T1)  [unwired: 2 in]
  }
  n375 = call-poly <vilib>:"PolyMotor.vi"("NXT"=w5, "Port (All Ports)"=w9) -> ("NXT"=w2:T1)  [unwired: 2 in]
  n376 = case shown="True" w1 {
    tunnel: w2 -> [w957 w962]
    tunnel: [w957 w959] -> _
    frame False {
    }
    frame True {
      w958 = T2 5 items=["Port A"=0, "Port B"=1, "Port C"=2, "Ports A & B"=4, "Ports A & C"=5, "Ports B & C"=6, "All Ports"=3] ("Output Port (All Ports)")
      # "robot is stuck"
      n377 = call-poly <vilib>:"PolySound.vi"("NXT"=w962) -> ("NXT"=w961:T1)  [unwired: 3 in]
      n378 = call <vilib>:"MotorDistance.vi"("Angle of Rotation (360)"=90, "NXT"=w961, "Output Port (All Ports)"=w958) -> ("NXT"=w959:T1)  [unwired: 1 in]
    }
  }
  "right(T)/left(F)" <- FALSE ("right(T)/left(F)")
